vi "前站查询(T1).vi"(6 "Station":string, 8 "Pre Check":bool, 9 "PN":string, 10 "DBSet":T1, 11 "SN":string) -> (3 "判定":bool)   [LabVIEW 2011]
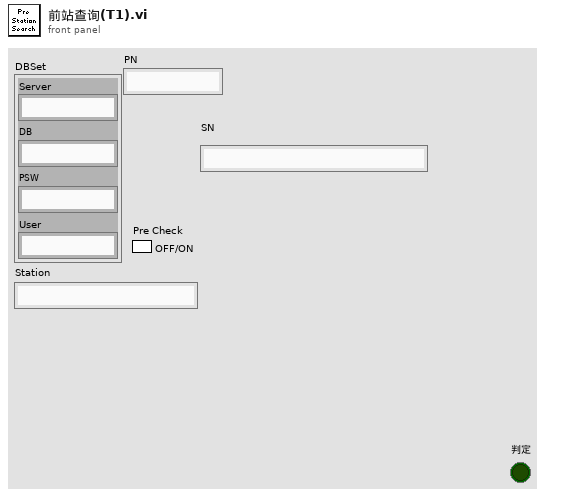
[diagram p1: front panel]
types:
  T1 = cluster{"Server":string, "DB":string, "PSW":string, "User":string}
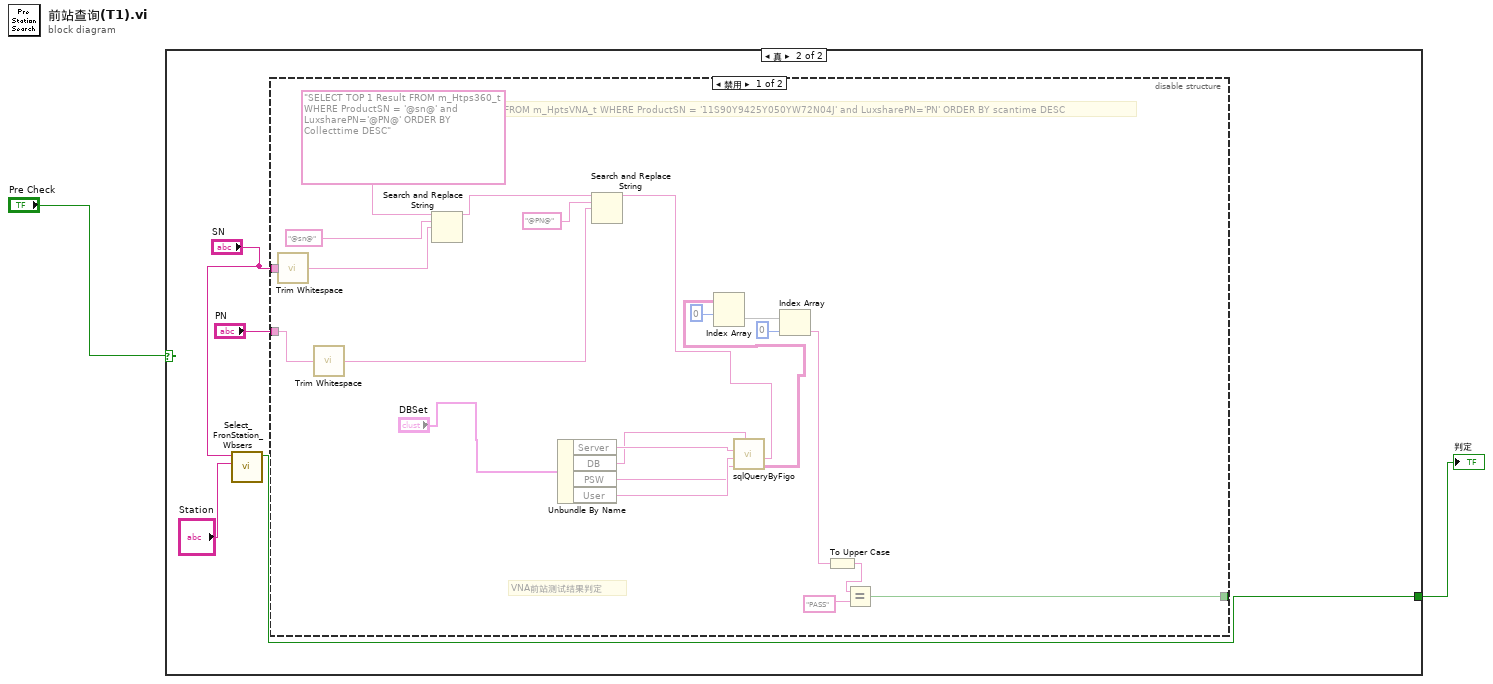
[diagram p0: block diagram]
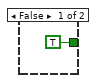
[diagram p2: hidden frame]
diagram:
  n1 = case shown="真" "Pre Check" {
    tunnel: [TRUE w5] -> w2
    frame False {
    }
    frame True {
      n2 = call "Select_FronStation_Wbsers.vi"("Station"="Station", "Barcode"="SN") -> ("GetCheckAssysDataResult"=w5:bool)  [unwired: 6 in, 3 out]
      n3 = disable-structure shown="禁用" {
        disable-tunnel: "SN" -> [w23 _]
        disable-tunnel: "PN" -> [w12 _]
        disable-tunnel: [w8 _] -> _
        frame Disabled {
          # "SELECT TOP 1 Result FROM m_HptsVNA_t WHERE ProductSN = '11S90Y9425Y050YW72N04J' and LuxsharePN='PN' ORDER BY scantime DESC"
          # "VNA前站测试结果判定"
          n4 = call <vilib>:"Trim Whitespace.vi"("string"=w23) -> ("trimmed string"=w22:string)  [unwired: 1 in]
          n5 = call <vilib>:"Trim Whitespace.vi"("string"=w12) -> ("trimmed string"=w11:string)  [unwired: 1 in]
          n6 = Search and Replace String(input string="SELECT TOP 1 Result FROM m_Htps360_t WHERE ProductSN = '@sn@' and LuxsharePN='@PN@' ORDER BY Collecttime DESC", search string="@sn@" ("搜索字符串"), replace string=w22) -> (result string=w15:string)  [unwired: 5 in, 3 out]
          n7 = Unbundle By Name("DBSet") -> ("Server"=w19:string, "DB"=w16:string, "PSW"=w17:string, "User"=w18:string)
          n8 = Search and Replace String(input string=w15, search string="@PN@" ("搜索字符串"), replace string=w11) -> (result string=w14:string)  [unwired: 5 in, 3 out]
          n9 = call "sqlQueryByFigo.vi"("SQL"=w14, "DATABASE"=w16, "password"=w17, "user id"=w18, "Server"=w19) -> ("查询数据"=w20:string[][])  [unwired: 5 in, 1 out]
          n10 = Index Array(array=w20, index (row)=0 ("索引 (行)")) -> (element=w26:string[])  [unwired: 1 in]
          n11 = Index Array(array=w26, index=0 ("索引")) -> (element=w10:string)
          n12 = To Upper Case(1:w10) -> (0:w9:string)
          n13 = Equal?(x=w9, y="PASS") -> (x = y?=w8:bool)
        }
        frame Enabled {
        }
      }
    }
  }
  "判定" <- w2
